vi "Open Thermometer Calib File.vi"() -> (0 "Byte Stream File Refnum":refnum<file>)   [LabVIEW 2020]
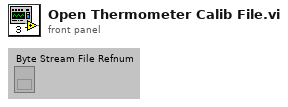
[diagram p1: front panel]
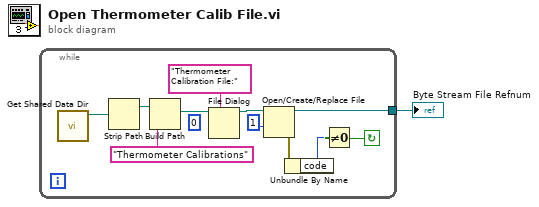
[diagram p0: block diagram]
diagram:
  n1 = while {
    tunnel: [w8] -> w1
    stop <- w7 continue-if-true
    (unwired) i16 0
    n2 = call "Get Shared Data Dir.vi"() -> ("Data Directory Path"=w5:path)  [unwired: 2 in, 1 out]
    n3 = Strip Path(path=w5) -> (stripped path=w2:path)  [unwired: 1 out]
    n4 = Build Path(base path=w2, name or relative path="Thermometer Calibrations") -> (appended path=w12:path)
    n5 = File Dialog(7:"Thermometer Calibration File:", 11:w12) -> (3:w9:path)  [unwired: 5 in, 3 out]
    n6 = Open/Create/Replace File(file path (use dialog)=w9, access (0:read/write)=i16 1) -> (refnum out=w8:refnum<file>, error out=w6:errorcluster)  [unwired: 4 in, 1 out]
    n7 = Unbundle By Name(w6) -> ("code"=w3:i32)
    n8 = Not Equal To 0?(x=w3) -> (x != 0?=w7:bool)
  }
  "Byte Stream File Refnum" <- w1
